vi "Config_HD_Read.vi"() -> (2 "Dev Address":T1)   [LabVIEW 2016]
uses:
  Hardware_DeviceAddresses.ctl
  MW_ctl_DeviceHandles..ctl
  <vilib>/Utility/config.llb/Read Key (String).vi
  Microwave Source.lvlib
  <vilib>/Utility/config.llb/NI_LVConfig.lvlib
panel:
  out "HardwareAddress.ini":path
  out "error out":errorcluster
  in  "error in (no error)":errorcluster
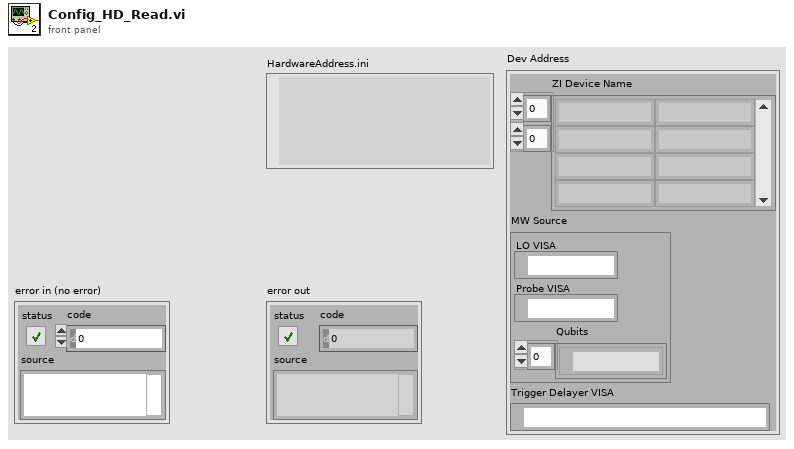
[diagram p1: front panel]
types:
  T1 = typedef "Hardware_DeviceAddresses.ctl" = cluster{"ZI Device Name":string[][], "MW Source":T2, "Trigger Delayer VISA":refnum<visa-resource-name>}
  T2 = typedef "Microwave Source.lvlib/MW_ctl_DeviceHandles..ctl" = cluster{"LO VISA":refnum<visa-resource-name>, "Probe VISA":refnum<visa-resource-name>, "Qubits":refnum<visa-resource-name>[]}
  T3 = typedef "Constant_FilePaths_ctl.ctl" = cluster{"Directories":cluster{"Application":path, "Config":path}, "Files":cluster{"HardwareAddress.ini":path}}
  T4 = typedef "NI_LVConfig.lvlib/Config Data RefNum.ctl" = refnum<k1>
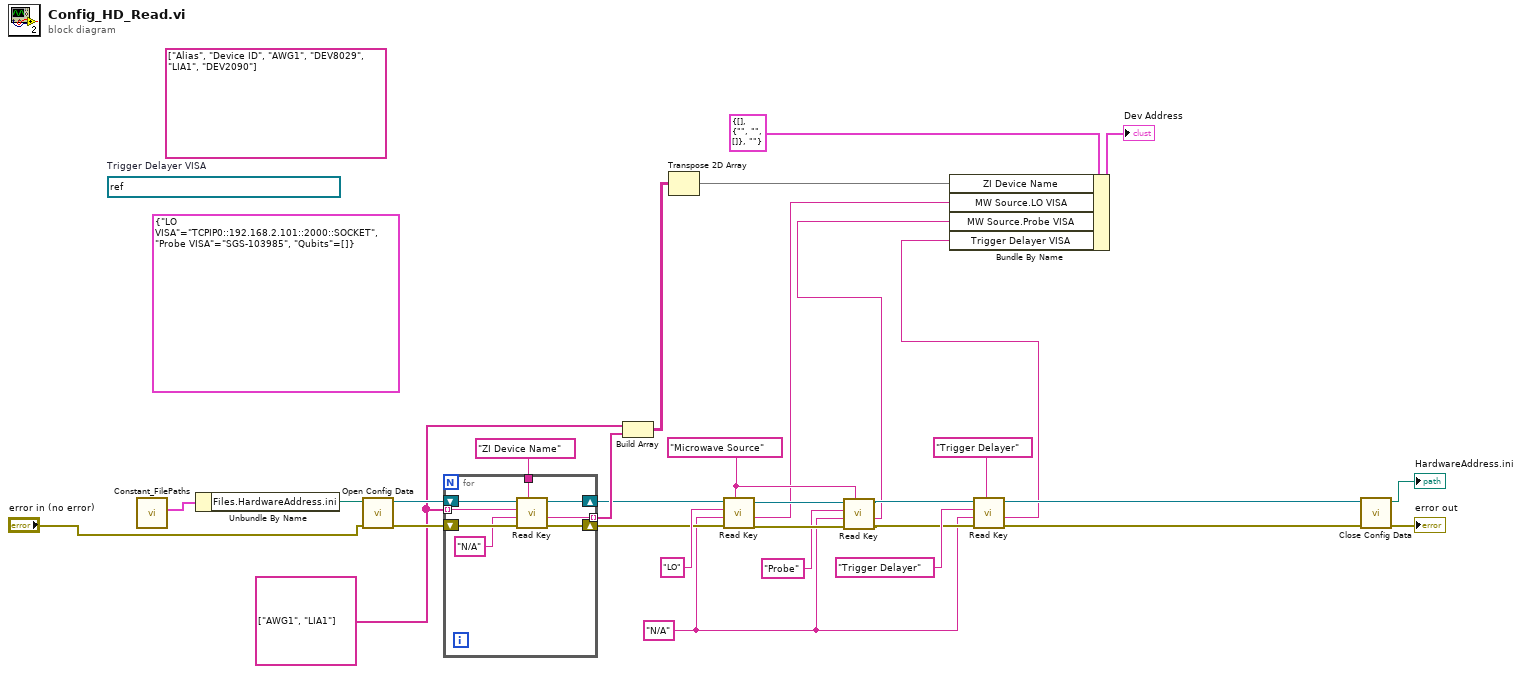
[diagram p0: block diagram]
diagram:
  w1 = "N/A" ("default value")
  w10 = string[] ["AWG1", "LIA1"]
  w30 = "Microwave Source" ("section")
  (unwired) refnum<visa-resource-name> "TCPIP0::192.168.2.10::5025::SOCKET"  # Trigger Delayer VISA
  (unwired) T2 {"LO VISA"="TCPIP0::192.168.2.101::2000::SOCKET", "Probe VISA"="SGS-103985", "Qubits"=[]} ("MW Source In")
  (unwired) string[][] [["Alias", "Device ID"], ["AWG1", "DEV8029"], ["LIA1", "DEV2090"]] ("Hardware Handle.Device Name")
  n1 = call "Constant_FilePaths.vi"() -> ("Paths"=w17:T3)  [unwired: 11 in]
  n2 = Unbundle By Name(w17) -> ("Files.HardwareAddress.ini"=w16:path)
  n3 = call <vilib>:"Open Config Data.vi"("error in (no error)"="error in (no error)", "configuration file path"=w16) -> ("error out"=w24:errorcluster, "refnum"=w25:T4)  [unwired: 7 in, 1 out]
  n4 = for {
    tunnel: "ZI Device Name" ("section") -> [w39]
    tunnel: w10 -> [w36] mode=indexing
    tunnel: [w34] -> w9 mode=indexing
    shift-right: [w33] -> w8
    shift-left: w25 -> [w38]
    shift-right: [w32] -> w7
    shift-left: w24 -> [w37]
    n5 = call-poly <vilib>:"Read Key.vi"("section"=w39, "error in (no error)"=w37, "default value"="N/A", "key"=w36, "refnum"=w38) -> ("error out"=w32:errorcluster, "value"=w34:string, "refnum out"=w33:T4)  [unwired: 3 in, 1 out]
  }
  n6 = Build Array(w10, w9) -> (w6:string[][])
  n7 = Transpose 2D Array(2D array=w6) -> (transposed array=w5:string[][])
  n8 = call-poly <vilib>:"Read Key.vi"("section"=w30, "error in (no error)"=w7, "default value"=w1, "key"="LO", "refnum"=w8) -> ("error out"=w28:errorcluster, "value"=w4:string, "refnum out"=w29:T4)  [unwired: 3 in, 1 out]
  n9 = call-poly <vilib>:"Read Key.vi"("section"=w30, "error in (no error)"=w28, "default value"=w1, "key"="Probe", "refnum"=w29) -> ("error out"=w21:errorcluster, "value"=w3:string, "refnum out"=w22:T4)  [unwired: 3 in, 1 out]
  n10 = call-poly <vilib>:"Read Key.vi"("section"="Trigger Delayer", "error in (no error)"=w21, "default value"=w1, "key"="Trigger Delayer", "refnum"=w22) -> ("error out"=w20:errorcluster, "value"=w2:string, "refnum out"=w19:T4)  [unwired: 3 in, 1 out]
  n11 = Bundle By Name(cluster=T1 {"ZI Device Name"=[], "MW Source"={"LO VISA"="", "Probe VISA"="", "Qubits"=[]}, "Trigger Delayer VISA"=""} ("Dev Add"), "ZI Device Name"=w5, "MW Source.LO VISA"=w4, "MW Source.Probe VISA"=w3, "Trigger Delayer VISA"=w2) -> (→"Dev Address":T1)
  n12 = call <vilib>:"Close Config Data.vi"("error in (no error)"=w20, "refnum"=w19) -> ("error out"=→"error out":errorcluster, "file path"=→"HardwareAddress.ini":path)  [unwired: 8 in]
